vi "Add Collection.vi"(8 "error in (no error)":errorcluster, 11 "Node Ptr":u64 format="%.0x") -> (0 "error out":errorcluster)   [LabVIEW 2024, in "Diagnostics Addon System Explorer.lvlib"]
uses:
  Diagnostics Addon System Explorer.lvlib
  Types/IO.Export.ctl
  Types/CmdResp.Export.ctl
  Addon Shared/Types/Signal.ctl
  Addon Shared/Types/Type.ctl
  Types/Routine.Export.ctl
  SubVIs/Name.Create.vi
  SubVIs/ID.FG.vi
  Addon Shared/SubVIs/Constants.vi
  <vilib>/NI/NI VeriStand Advanced SysDef API/SysDef API/SysDef.CreateSection.vi
  <vilib>/NI/NI VeriStand Advanced SysDef API/SysDef API/SysDef.Property.Set.vi
  <vilib>/NI/NI VeriStand Advanced SysDef API/_SubVIs/SysDef.Property.Set.U32.vi
  <vilib>/NI VeriStand/Custom Device API/NI VeriStand - Get Item Property.vi
  <vilib>/NI VeriStand/Custom Device API/Get Item Property (U32).vi
  <vilib>/NI VeriStand/Custom Device API/Custom Device API.lvlib
  <vilib>/NI VeriStand/Custom Device Tools/Custom Device Utility Library/Custom Device Utility Library.lvlib
  Addon Shared/Diagnostics Addon Shared.lvlib
panel:
  in  "Tag":string
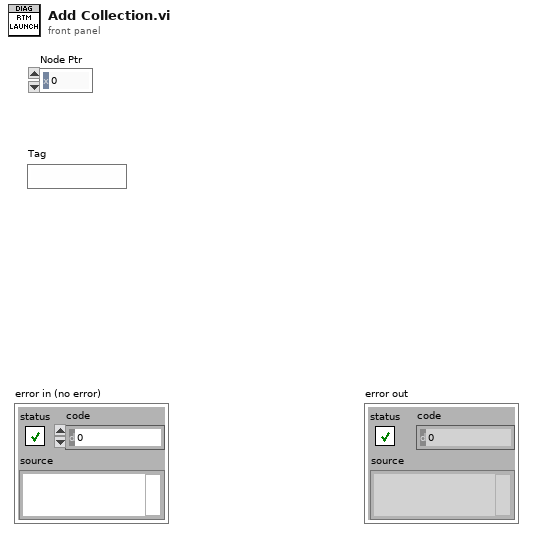
[diagram p1: front panel]
types:
  T1 = typedef "Custom Device API.lvlib/Custom Device Item Info.ctl" = cluster{"Name":string, "Is Channel":bool, "GUID":string, "Is Waveform":bool}
  T2 = typedef "Custom Device API.lvlib/Custom Device Item Ref.ctl" = u64
  T3 = typedef "Diagnostics Addon Shared.lvlib/Type.ctl" = enum16{"DID", "CDID", "PID", "CPID", "Read Memory", "Write Memory", "IO Control", "Routine Start", "Routine Request", "Routine Stop", "User Defined", "DTC Control", "Clear DTCs", "Read DTCs", "Start DTCs", "DTC Change Count", "Tester Present", "Unlock ECU", "Reset ECU", "Diag Session Control", "Communication Control", "DPID Control", "Poll Control", "Diag Comm Port Control"}
  T4 = typedef "Diagnostics Addon System Explorer.lvlib/IO.Export.ctl" = cluster{"Name":string, "ID":u16, "Signals":T5}
  T5 = typedef "Diagnostics Addon System Explorer.lvlib/CmdResp.Export.ctl" = cluster{"Cmd":T6[], "Response":T6[]}
  T6 = typedef "Diagnostics Addon Shared.lvlib/Signal.ctl" = cluster{"Start Bit":u32, "Length":u32, "Scaling Factor":dbl, "Scaling Offset":dbl, "Minimum":dbl, "Maximum":dbl, "Data Type":u32, "Byte Order":u32, "Default Value":dbl, "Name":string, "Units":string}
  T7 = typedef "Diagnostics Addon System Explorer.lvlib/Routine.Export.ctl" = cluster{"Name":string, "ID":u16, "Start Parameters":T5, "Request Parameters":T5, "Stop Parameters":T5}
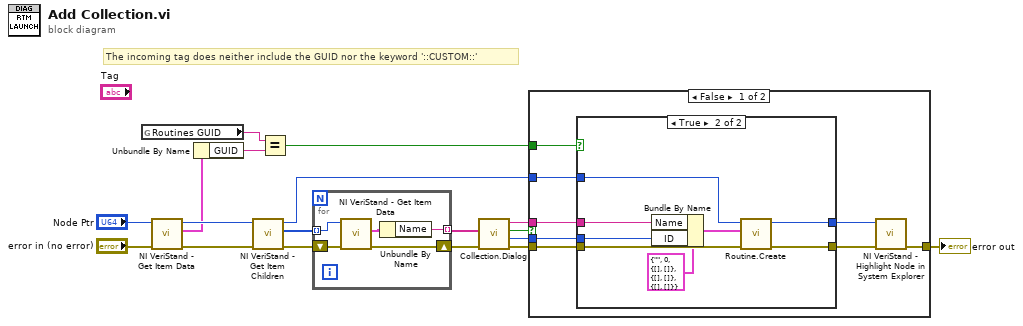
[diagram p0: block diagram]
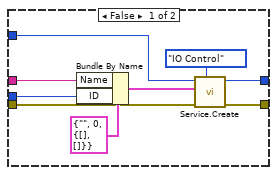
[diagram p2: hidden frame]
diagram:
  # "The incoming tag does neither include the GUID nor the keyword '::CUSTOM::'"
  n1 = global read "Constants.vi" "Routines GUID"() -> (w2:string)
  n2 = call <vilib>:"NI VeriStand - Get Item Data.vi"("error in (no error)"="error in (no error)", "Item Ref in"="Node Ptr") -> ("error out"=w7:errorcluster, "Item Info"=w4:T1, "Item Ref out"=w6:T2)  [unwired: 7 out]
  n3 = Unbundle By Name(w4) -> ("GUID"=w3:string)
  n4 = call <vilib>:"NI VeriStand - Get Item Children.vi"("error in (no error)"=w7, "Item Ref in"=w6) -> ("error out"=w18:errorcluster, "Child Refs"=w16:T2[], "Item Ref out"=w15:T2)  [unwired: 6 in, 1 out]
  n5 = Equal?(x=w2, y=w3) -> (x = y?=w1:bool)
  n6 = for {
    tunnel: [w21] -> w14 mode=indexing
    shift-right: [w20] -> w13
    shift-left: w18 -> [w22]
    tunnel: w16 -> [w19] mode=indexing
    n7 = call <vilib>:"NI VeriStand - Get Item Data.vi"("error in (no error)"=w22, "Item Ref in"=w19) -> ("error out"=w20:errorcluster, "Item Info"=w23:T1)  [unwired: 8 out]
    n8 = Unbundle By Name(w23) -> ("Name"=w21:string)
  }
  n9 = call "Collection.Dialog.vi"("error in (no error)"=w13, "Existing PIDs"=w14) -> ("error out"=w12:errorcluster, "ID out"=w11:u16, "Cancel PID?"=w10:bool, "Name out"=w9:string)  [unwired: 6 in]
  n10 = case shown="False" w10 {
    tunnel: w12 -> [w30 w49]
    tunnel: w15 -> [w27 _]
    tunnel: w9 -> [w26 _]
    tunnel: [w31 w49] -> w17
    tunnel: w11 -> [w25 _]
    tunnel: w1 -> [w24 _]
    frame False {
      n11 = case shown="True" w24 {
        tunnel: w30 -> [w34 w48]
        tunnel: [w33 w47] -> w29
        tunnel: [w35 w46] -> w28
        tunnel: w27 -> [w36 w45]
        tunnel: w26 -> [w40 w42]
        tunnel: w25 -> [w39 w41]
        frame False {
          n12 = Bundle By Name(cluster=T4 {"Name"="", "ID"=0, "Signals"={"Cmd"=[], "Response"=[]}} ("IO Control"), "Name"=w40, "ID"=w39) -> (w37:T4)
          n13 = call "Service.Create.vi"("Type"=Type."IO Control", "error in (no error)"=w34, "Variant"=w37, "Section Ptr"=w36) -> ("error out"=w33:errorcluster, "Parent Ref out"=w35:T2)  [unwired: 6 in]
        }
        frame True {
          n14 = Bundle By Name(cluster=T7 {"Name"="", "ID"=0, "Start Parameters"={"Cmd"=[], "Response"=[]}, "Request Parameters"={"Cmd"=[], "Response"=[]}, "Stop Parameters"={"Cmd"=[], "Response"=[]}} ("Routine"), "Name"=w42, "ID"=w41) -> (w43:T7)
          n15 = call "Routine.Create.vi"("error in (no error)"=w48, "Routine"=w43, "Section Ptr"=w45) -> ("error out"=w47:errorcluster, "Parent Ref out"=w46:T2)  [unwired: 7 in]
        }
      }
      n16 = call <vilib>:"NI VeriStand - Highlight Node in System Explorer.vi"("error in (no error)"=w29, "Item Ref in"=w28) -> ("error out"=w31:errorcluster)  [unwired: 8 in, 1 out]
    }
    frame True {
    }
  }
  "error out" <- w17
